vi "UMM_Admin.vi"(8 "error in (no error)":errorcluster caption="错误输入（无错误）", 11 "User Management Model 输入":refnum<class "User Management Model.lvclass">) -> (0 "error out":errorcluster caption="错误输出", 2 "信息显示":string[][](table), 3 "User Management Model 输出":refnum<class "User Management Model.lvclass">)   [LabVIEW 2019, in "User Management Model.lvclass"]
uses:
  User Management Model.lvclass
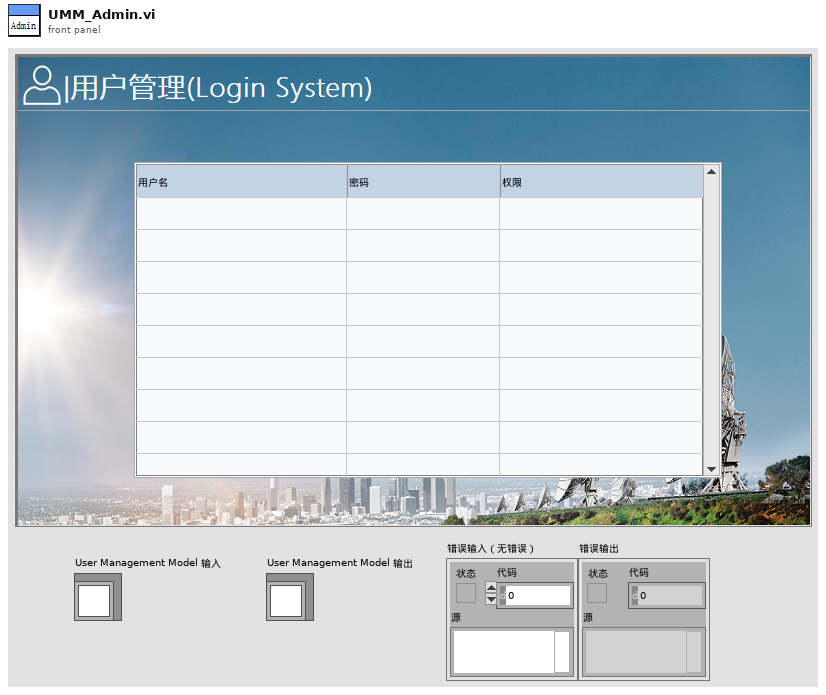
[diagram p1: front panel]
types:
  T1 = enum16{"open", "replace", "create", "open or create", "replace or create", "replace or create with confirmation"}
  T2 = typedef "LVPoint32TypeDef.ctl" = cluster{"Horizontal":i32, "Vertical":i32}
  T3 = typedef "LVRowAndColumnTypeDef.ctl" = cluster{"Row":i32, "Column":i32}
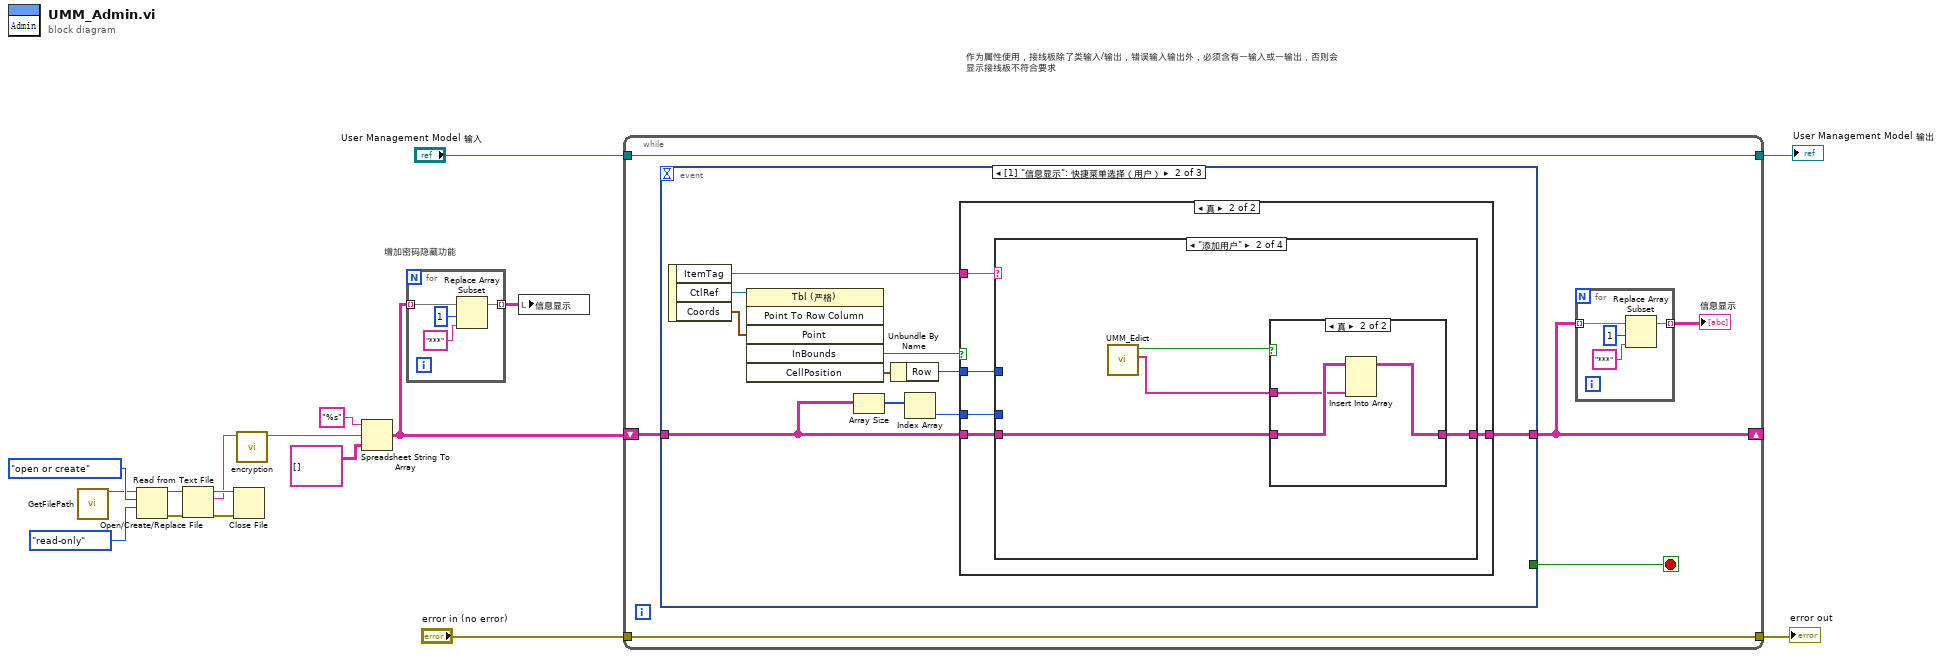
[diagram p0: block diagram]
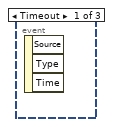
[diagram p2: hidden frame]
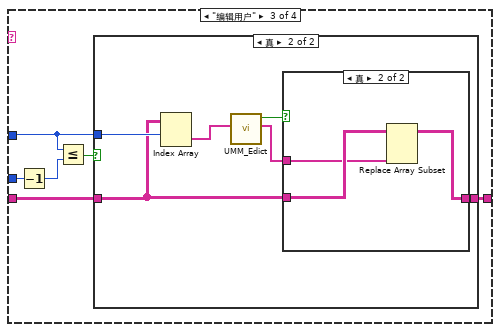
[diagram p6: hidden frame]
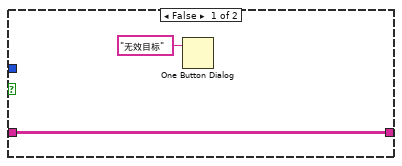
[diagram p7: hidden frame]
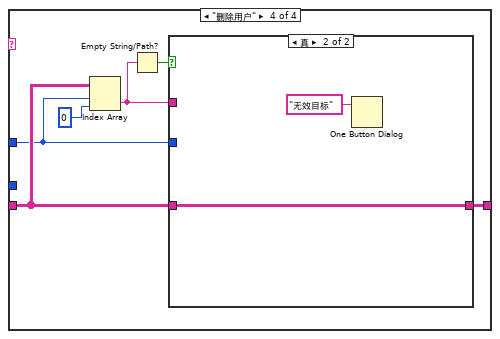
[diagram p9: hidden frame]
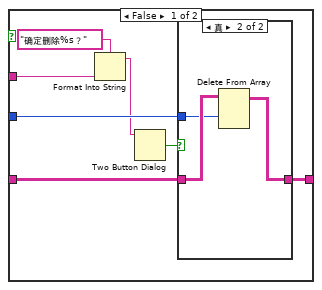
[diagram p10: hidden frame]
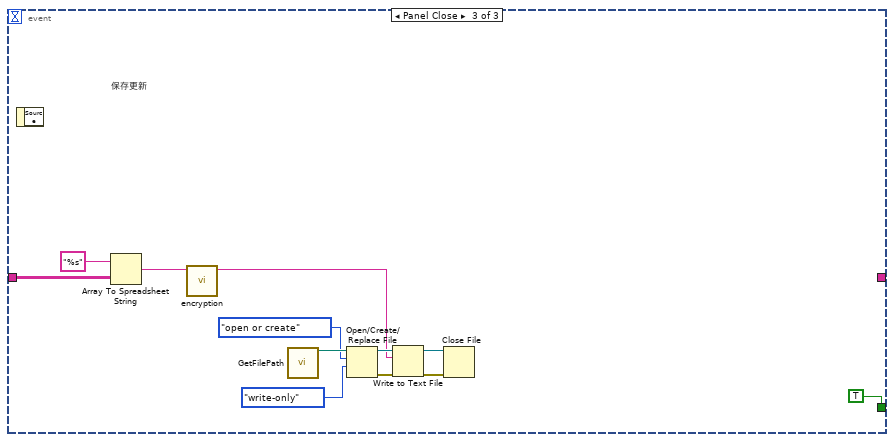
[diagram p12: hidden frame]
diagram:
  # "作为属性使用，接线板除了类输入/输出，错误输入输出外，必须含有一输入或一输出，否则会\n显示接线板不符合要求"
  # "增加密码隐藏功能"
  n1 = call "GetFilePath.vi"() -> ("添加的路径"=w12:path)  [unwired: 19 in]
  n2 = Open/Create/Replace File(file path (use dialog)=w12, operation (0:open)=T1."open or create" ("操作(0:open)"), access (0:read/write)=enum16{"read/write", "read-only", "write-only"}."read-only" ("权限(0:read/write)")) -> (refnum out=w16:refnum<file>, error out=w15:errorcluster)  [unwired: 3 in, 1 out]
  n3 = Read from Text File(file (use dialog)=w16, error in=w15) -> (refnum out=w14:refnum<file>, text=w11:string, error out=w13:errorcluster)  [unwired: 2 in, 1 out]
  n4 = Close File(refnum=w14, error in=w13) -> ()  [unwired: 2 out]
  n5 = call "encryption.vi"("字符串"=w11) -> ("转换值"=w10:string)  [unwired: 10 in]
  n6 = Spreadsheet String To Array(format string="%s" ("格式字符串"), spreadsheet string=w10, array type (2D Dbl)=string[][] [] ("格式字符串")) -> (array=w7:string[][])  [unwired: 1 in]
  n7 = for {
    tunnel: w7 -> [w21] mode=indexing
    tunnel: [w18] -> w6 mode=indexing
    n8 = Replace Array Subset(array=w21, new element="***" ("新元素/子数组"), index=1 ("索引")) -> (w18:string[])
  }
  n9 = local write "信息显示"(w6) -> ()
  n10 = while {
    shift-right: [w25] -> _
    shift-left: w7 -> [w27]
    tunnel: "User Management Model 输入" -> [w22]
    tunnel: "error in (no error)" -> [w23]
    tunnel: [w23] -> w2
    tunnel: [w22] -> w1
    stop <- w26 stop-if-true
    n11 = event shown="[1] \"信息显示\": 快捷菜单选择（用户）" {
      selector: _ -> [_ _ _]
      dyn-events: _ -> [_ _ _]
      timeout: _ -> [_ _ _]
      tunnel: w27 -> [_ w34 w104]
      tunnel: [_ w36 _] -> w25
      tunnel: [_ _ TRUE] -> w26
      event Timeout {
        n12 = event-data() -> ()  [unwired: 1 in, 3 out]
      }
      event "信息显示": Shortcut Menu Selection (User) {
        n13 = event-data() -> ("ItemTag"=w37:string, "CtlRef"=w41:refnum<vi>, "Coords"=w40:T2)  [unwired: 1 in]
        n14 = invoke class="Tbl (严格)" method="Point To Row Column"(reference=w41, "Point"=w40) -> ("InBounds"=w38:bool, "CellPosition"=w39:T3)  [unwired: 4 in, 4 out]
        n15 = Array Size(array=w34) -> (size(s)=w33:i32[])
        n16 = Unbundle By Name(w39) -> ("Row"=w35:i32)
        n17 = Index Array(array=w33) -> (element=w32:i32)  [unwired: 1 in]
        n18 = case shown="真" w38 {
          tunnel: w37 -> [_ w47]
          tunnel: w34 -> [w42 w46]
          tunnel: [w42 w45] -> w36
          tunnel: w35 -> [_ w44]
          tunnel: w32 -> [_ w43]
          frame False {
          }
          frame True {
            n19 = case shown="\"添加用户\"" w47 {
              tunnel: w46 -> [w48 w52 w62 w79]
              tunnel: [w48 w51 w61 w80] -> w45
              tunnel: w44 -> [_ _ w60 w78]
              tunnel: w43 -> [_ _ w58 _]
              frame Default {
              }
              frame "添加用户" {
                n20 = call "UMM_Edict.vi"() -> ("信息 out"=w49:string[], "sure？"=w50:bool)  [unwired: 10 in]
                n21 = case shown="真" w50 {
                  tunnel: w52 -> [w53 w56]
                  tunnel: [w53 w55] -> w51
                  tunnel: w49 -> [_ w54]
                  frame False {
                  }
                  frame True {
                    n22 = Insert Into Array(array=w56, new element=w54) -> (w55:string[][])  [unwired: 2 in]
                  }
                }
              }
              frame "编辑用户" {
                n23 = Decrement(x=w58) -> (x-1=w57:i32)
                n24 = Less Or Equal?(x=w60, y=w57) -> (x <= y?=w59:bool)
                n25 = case shown="真" w59 {
                  tunnel: w60 -> [_ w70]
                  tunnel: w62 -> [w63 w69]
                  tunnel: [w63 w68] -> w61
                  frame False {
                    n26 = One Button Dialog(message="无效目标" ("消息")) -> ()  [unwired: 1 in, 1 out]
                  }
                  frame True {
                    n27 = Index Array(array=w69, index (row)=w70) -> (element=w66:string[])  [unwired: 1 in]
                    n28 = call "UMM_Edict.vi"("信息"=w66) -> ("信息 out"=w65:string[], "sure？"=w67:bool)  [unwired: 9 in]
                    n29 = case shown="真" w67 {
                      tunnel: w69 -> [w71 w74]
                      tunnel: [w71 w73] -> w68
                      tunnel: w65 -> [_ w72]
                      frame False {
                      }
                      frame True {
                        n30 = Replace Array Subset(array=w74, new element=w72) -> (w73:string[][])  [unwired: 2 in]
                      }
                    }
                  }
                }
              }
              frame "删除用户" {
                n31 = Index Array(array=w79, index (row)=w78, index (col)=0 ("禁用的索引 (列)")) -> (element=w76:string)
                n32 = Empty String/Path?(string/path=w76) -> (empty?=w75:bool)
                n33 = case shown="真" w75 {
                  tunnel: [w87 w93] -> w80
                  tunnel: w79 -> [w85 w93]
                  tunnel: w78 -> [w84 _]
                  tunnel: w76 -> [w81 _]
                  frame False {
                    n34 = Format Into String(format string="确定删除%s？" ("消息"), w81) -> (resulting string=w82:string)  [unwired: 2 in, 1 out]
                    n35 = Two Button Dialog(message=w82) -> (T button?=w86:bool)  [unwired: 2 in]
                    n36 = case shown="真" w86 {
                      tunnel: w85 -> [w88 w91]
                      tunnel: w84 -> [_ w90]
                      tunnel: [w88 w89] -> w87
                      frame False {
                      }
                      frame True {
                        n37 = Delete From Array(array=w91, index (row)=w90) -> (array with subset deleted=w89:string[][])  [unwired: 2 in, 1 out]
                      }
                    }
                  }
                  frame True {
                    n38 = One Button Dialog(message="无效目标" ("消息")) -> ()  [unwired: 1 in, 1 out]
                  }
                }
              }
            }
          }
        }
      }
      event Panel Close {
        # "保存更新"
        n39 = event-data() -> ()  [unwired: 1 in, 1 out]
        n40 = Array To Spreadsheet String(array=w104, 3:"%s" ("格式字符串")) -> (spreadsheet string=w102:string)  [unwired: 1 in]
        n41 = call "encryption.vi"("字符串"=w102) -> ("转换值"=w94:string)  [unwired: 10 in]
        n42 = call "GetFilePath.vi"() -> ("添加的路径"=w101:path)  [unwired: 19 in]
        n43 = Open/Create/Replace File(file path (use dialog)=w101, operation (0:open)=T1."open or create" ("操作(0:open)"), access (0:read/write)=enum16{"read/write", "read-only", "write-only"}."write-only" ("权限(0:read/write)")) -> (refnum out=w97:refnum<file>, error out=w98:errorcluster)  [unwired: 3 in, 1 out]
        n44 = Write to Text File(file (use dialog)=w97, text=w94, error in=w98) -> (refnum out=w99:refnum<file>, error out=w100:errorcluster)  [unwired: 1 in, 1 out]
        n45 = Close File(refnum=w99, error in=w100) -> ()  [unwired: 2 out]
      }
    }
    n46 = for {
      tunnel: w25 -> [w31] mode=indexing
      tunnel: [w28] -> w24 mode=indexing
      n47 = Replace Array Subset(array=w31, new element="***" ("新元素/子数组"), index=1 ("索引")) -> (w28:string[])
    }
    "信息显示" <- w24
  }
  "error out" <- w2
  "User Management Model 输出" <- w1
